vi "Add and sub.vi"(9 "B":dbl, 10 "A":dbl) -> (1 "A - B":dbl, 2 "A + B":dbl)   [LabVIEW 2014]
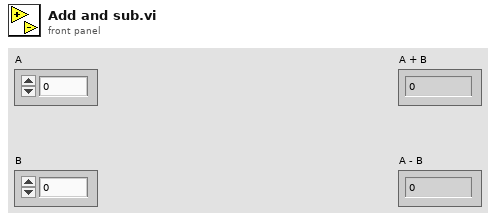
[diagram p1: front panel]
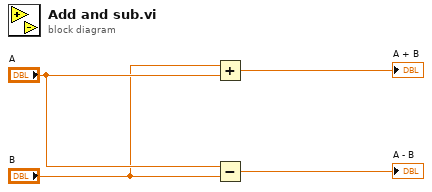
[diagram p0: block diagram]
diagram:
  n1 = Add(x="B", y="A") -> (x+y=→"A + B":dbl)
  n2 = Subtract(x="A", y="B") -> (x-y=→"A - B":dbl)
